vi "Untitled 1.vi"() -> ()   [LabVIEW 2011]
panel:
  in  "Breake":bool
  in  "Acelerador":bool
  in  "on/off Auto":bool
  out "VELOCIDAD":i32(knob) scale=1.0..220.0
  # "Generar la velocidad del auto entre 1-20 y luego debemos de presionar el\n acelerador para aumentar la velocidad en 10 y presionar  el breake para disminuir a 5"
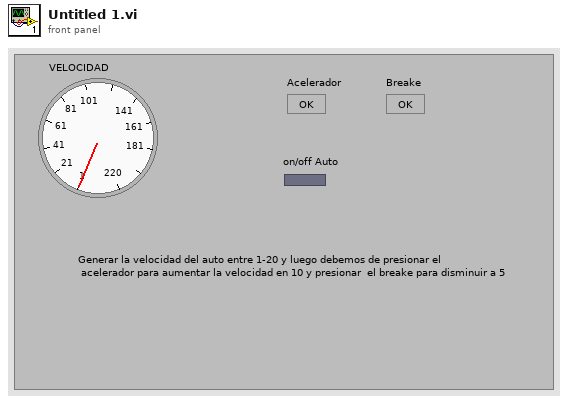
[diagram p1: front panel]
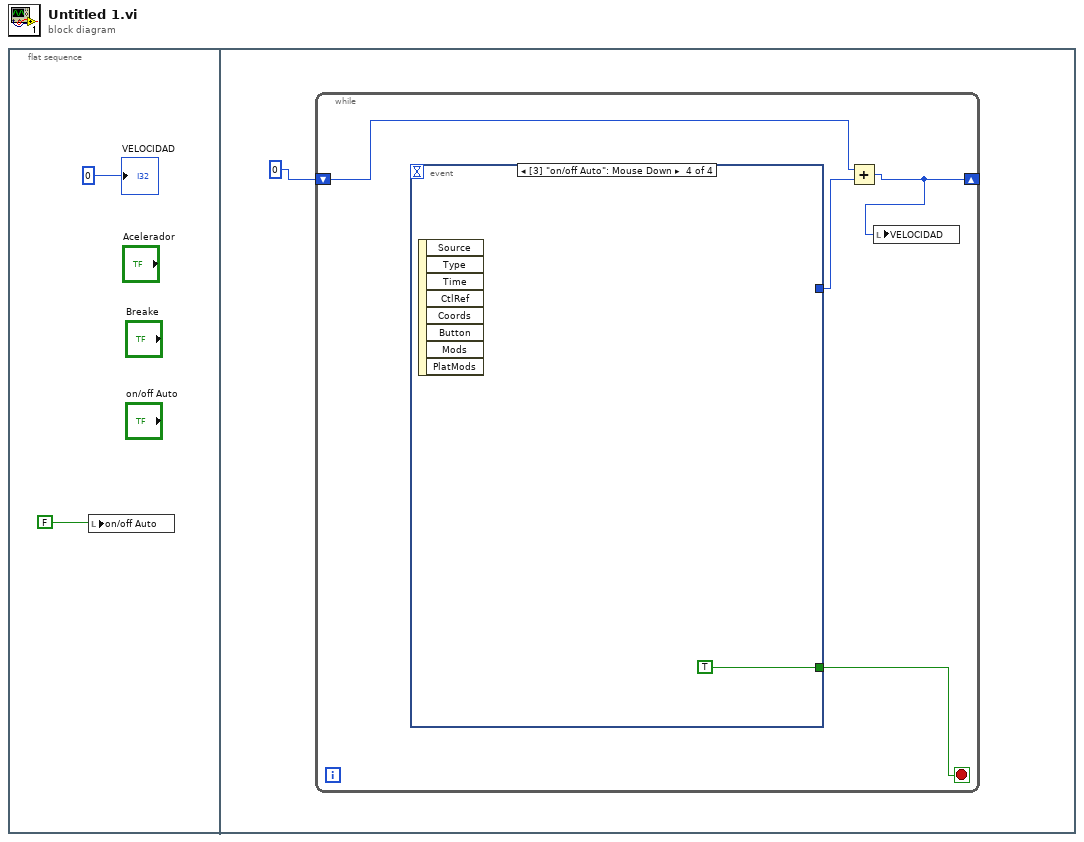
[diagram p0: block diagram]
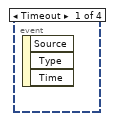
[diagram p2: hidden frame]
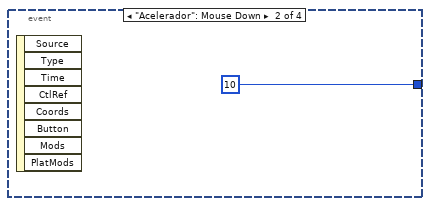
[diagram p3: hidden frame]
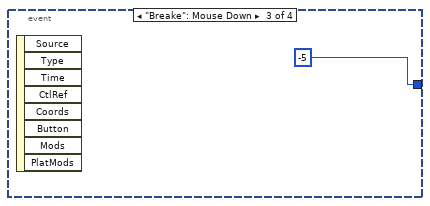
[diagram p4: hidden frame]
diagram:
  n1 = flat-sequence {
    frame #0 {
      n2 = local write "on/off Auto"(FALSE) -> ()
      "VELOCIDAD" <- 0
    }
    frame #1 {
      n3 = while {
        shift-right: [w5] -> _
        shift-left: 0 -> [w7]
        stop <- w4 stop-if-true
        n4 = event shown="[3] \"on/off Auto\": Mouse Down" {
          selector: _ -> [_ _ _ _]
          dyn-events: _ -> [_ _ _ _]
          timeout: _ -> [_ _ _ _]
          tunnel: [_ 10 -5 _] -> w6
          tunnel: [_ _ _ TRUE] -> w4
          event Timeout {
            n5 = event-data() -> ()  [unwired: 1 in, 3 out]
          }
          event "Acelerador": Mouse Down {
            n6 = event-data() -> ()  [unwired: 1 in, 8 out]
          }
          event "Breake": Mouse Down {
            n7 = event-data() -> ()  [unwired: 1 in, 8 out]
          }
          event "on/off Auto": Mouse Down {
            n8 = event-data() -> ()  [unwired: 1 in, 8 out]
          }
        }
        n9 = Add(x=w7, y=w6) -> (x+y=w5:i32)
        n10 = local write "VELOCIDAD"(w5) -> ()
      }
    }
  }
